vi "VG-Fill_Com_ports.vi"() -> (2 "output cluster":T1={"Com"="", "baud rate (9600)"=38400} {"baud rate (9600)" items=["75"=75, "110"=110, "134"=134, "150"=150, "300"=300, "600"=600, "1200"=1200, "1800"=1800, "2400"=2400, "4800"=4800, "7200"=7200, "9600"=9600, "14400"=14400, "19200"=19200, "28800"=28800, "38400"=38400, "56000"=56000, "57600"=57600, "115200"=115200, "128000"=128000, "230400"=230400]})   [LabVIEW 2020, in "VG-VNA_GUI.lvlib" / "VG-VNA_GUI.lvclass"]
uses:
  VG-VNA_GUI.lvclass
  classes/vna-drivers/liteVNA/VD-connection_settings.ctl
  classes/hardware-protocol/serial/HP-S-baudrate.ctl
  <vilib>/Instr/_visa.llb/VISA Find Search Mode.ctl
  classes/hardware-protocol/serial/HP-S-Serial.lvclass
  classes/vna-drivers/liteVNA/VD-LV-LiteVNA.lvclass
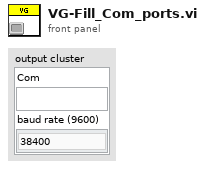
[diagram p1: front panel]
types:
  T1 = typedef "VD-LV-LiteVNA.lvclass/VD-connection_settings.ctl" = cluster{"Com":refnum<visa-resource-name>, "baud rate (9600)":T2}
  T2 = typedef "HP-S-Serial.lvclass/HP-S-baudrate.ctl" = u32
  T3 = typedef "VISA Find Search Mode.ctl" = u32
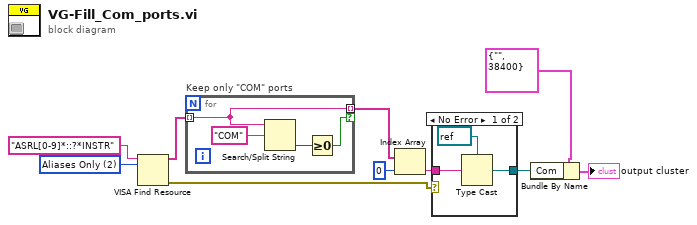
[diagram p0: block diagram]
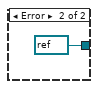
[diagram p2: hidden frame]
diagram:
  w8 = T3 2 items=["Canonical Names Only"=0, "Aliases Only"=2, "Include Matching Aliases"=3, "Include All Aliases"=4] ("Search Mode")
  n1 = VISA Find Resource(10:w8, 11:"ASRL[0-9]*::?*INSTR" ("expression (\"?*\")")) -> (0:w4:errorcluster, 3:w10:string[])  [unwired: 1 in, 1 out]
  n2 = for "Keep only \"COM\" ports" {
    tunnel: w10 -> [w12] mode=indexing
    tunnel: [w12] -> w7 mode=indexing if=w11
    n3 = Search/Split String(string=w12, search string/char (-)="COM") -> (offset of match=w13:i32)  [unwired: 1 in, 2 out]
    n4 = Greater Or Equal To 0?(x=w13) -> (x >= 0?=w11:bool)
  }
  n5 = Index Array(array=w7, index=0) -> (element=w5:string)
  n6 = case shown="No Error" w4 {
    tunnel: w5 -> [w16 _]
    tunnel: [w15 refnum<visa-resource-name> refnum ("Com")] -> w2
    frame No Error {
      n7 = Type Cast(type=refnum<visa-resource-name> refnum ("Com"), x=w16) -> (*(type *) &x=w15:refnum<visa-resource-name>)
    }
    frame Error {
    }
  }
  n8 = Bundle By Name(cluster=T1 {"Com"="", "baud rate (9600)"=38400} ("connection settings"), "Com"=w2) -> (→"output cluster":T1)
